vi "fuzzy_pid.vi"() -> ()   [LabVIEW 2019]
uses:
  <vilib>/addons/Fuzzy Logic/FL Fuzzy Controller (SISO).vi
  <vilib>/addons/Fuzzy Logic/NI_Fuzzy_Logic_API.lvlib
panel:
  in  "file path q2":path
  in  "file path q1":path
  out "Waveform Chart":T1(graph)
  in  "Set point":dbl
  in  "file path q0":path
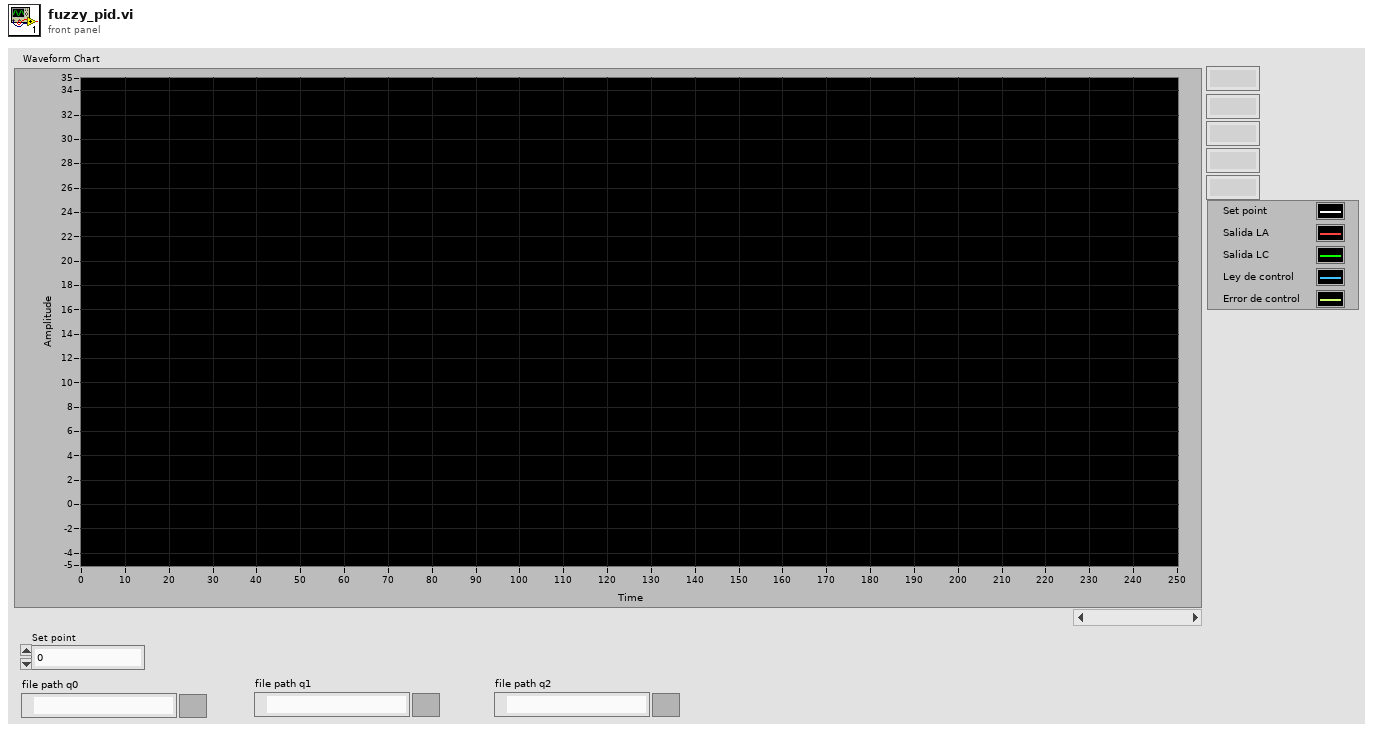
[diagram p1: front panel]
types:
  T1 = cluster{"Valvula (u_k)":dbl, "y_k":dbl, "y_k":dbl, dbl, dbl}
  T2 = typedef "NI_Fuzzy_Logic_API.lvlib/FL System.ctl" = cluster{"input variables":T3[], "output variables":T3[], "rules":T6[], "defuzzification method":T12, "description":string, "user MF interpolating polynomials":T13[]}
  T3 = typedef "NI_Fuzzy_Logic_API.lvlib/FL Variable.ctl" = cluster{"name":string, "range":dbl[], "MFs":T4[]}
  T4 = typedef "NI_Fuzzy_Logic_API.lvlib/FL Membership Function.ctl" = cluster{"name":string, "shape":T5, "points":dbl[], "color":u32, "user-defined shape index":i32}
  T5 = typedef "NI_Fuzzy_Logic_API.lvlib/FL Membership Function Shape.ctl" = u16
  T6 = typedef "NI_Fuzzy_Logic_API.lvlib/FL Rule.ctl" = cluster{"antecedents":T7[], "antecedent connective":T9, "consequents":T10[], "consequent implication":T11, "degree of support":dbl}
  T7 = typedef "NI_Fuzzy_Logic_API.lvlib/FL Antecedent.ctl" = cluster{"Var Index":i32, "MF Index":i32, "Cond":T8}
  T8 = typedef "NI_Fuzzy_Logic_API.lvlib/FL Modifier.ctl" = u16
  T9 = typedef "NI_Fuzzy_Logic_API.lvlib/FL Antecedent Connective.ctl" = u16
  T10 = typedef "NI_Fuzzy_Logic_API.lvlib/FL Consequent.ctl" = cluster{"Var Index":i32, "MF Index":i32, "Cond":T8}
  T11 = typedef "NI_Fuzzy_Logic_API.lvlib/FL Consequent Implication.ctl" = u16
  T12 = typedef "NI_Fuzzy_Logic_API.lvlib/FL Defuzzification.ctl" = u16
  T13 = typedef "NI_Fuzzy_Logic_API.lvlib/FL Interpolating polynomials.ctl" = cluster{"X":dbl[], "Y":dbl[], "Y(x) coeff":dbl[][], "X(y) coeff":dbl[][], "Area(y) coeff":dbl[][], "coa_x(y) coeff":dbl[][]}
  T14 = cluster{"Set point":dbl, "y_k":dbl, "y_k":dbl, dbl, dbl}
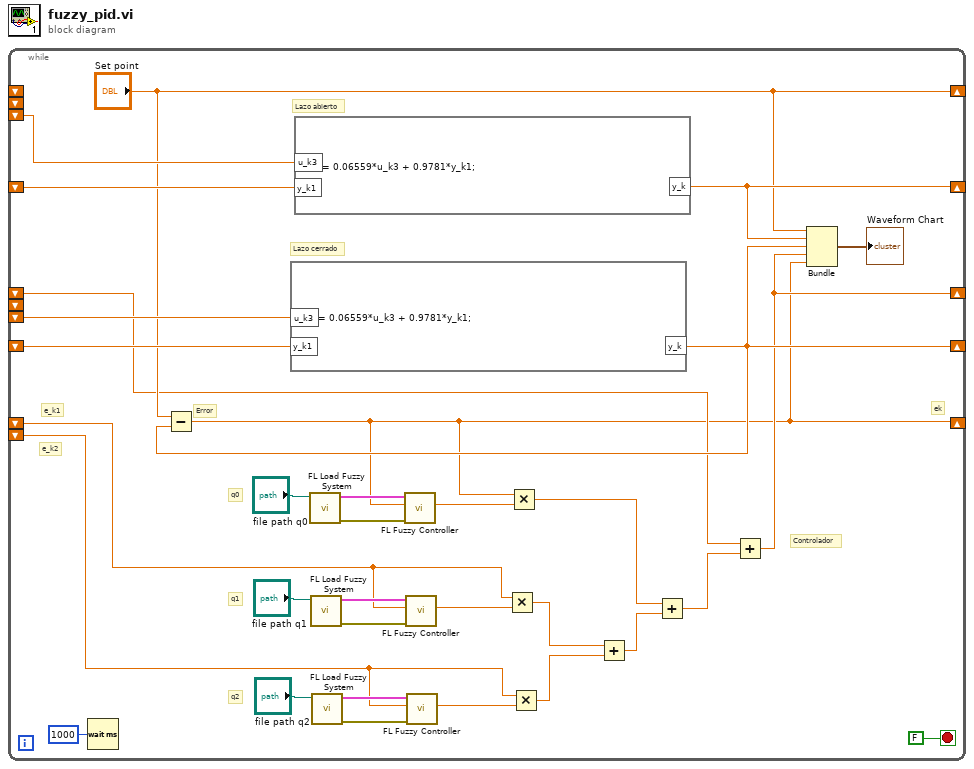
[diagram p0: block diagram]
diagram:
  n1 = while {
    shift-right: ["Set point"] -> _
    shift-left: _ -> [_]
    shift-left: _ -> [_]
    shift-left: _ -> [w32]
    shift-right: [w29] -> _
    shift-left: _ -> [w31]
    shift-right: [w21] -> _
    shift-left: _ -> [w24]
    shift-right: [w3] -> _
    shift-left: _ -> [w2]
    shift-left: _ -> [_]
    shift-left: _ -> [w23]
    shift-right: [w1] -> _
    shift-left: _ -> [w6]
    shift-left: _ -> [w5]
    stop <- FALSE stop-if-true
    # "Lazo cerrado"
    # "Lazo abierto"
    # "e_k2"
    # "e_k1"
    # "ek"
    # "Controlador"
    # "q2"
    # "q1"
    # "q0"
    # "Error"
    n2 = Wait (ms)(milliseconds to wait=u32 1000) -> ()  [unwired: 1 out]
    n3 = formula code="y_k = 0.06559*u_k3 + 0.9781*y_k1;"("u_k3"=w23, "y_k1"=w24) -> ("y_k"=w21:dbl)
    n4 = Subtract(x="Set point", y=w21) -> (x-y=w1:dbl)
    n5 = formula code="y_k = 0.06559*u_k3 + 0.9781*y_k1;"("u_k3"=w32, "y_k1"=w31) -> ("y_k"=w29:dbl)
    n6 = call <vilib>:"FL Load Fuzzy System.vi"("file path"="file path q0") -> ("error out"=w25:errorcluster, "fuzzy system out"=w26:T2)  [unwired: 9 in]
    n7 = call <vilib>:"FL Load Fuzzy System.vi"("file path"="file path q1") -> ("error out"=w18:errorcluster, "fuzzy system out"=w19:T2)  [unwired: 9 in]
    n8 = call <vilib>:"FL Load Fuzzy System.vi"("file path"="file path q2") -> ("error out"=w15:errorcluster, "fuzzy system out"=w16:T2)  [unwired: 9 in]
    n9 = call-poly <vilib>:"FL Fuzzy Controller.vi"("error in (no error)"=w25, "input value"=w1, "fuzzy system in"=w26) -> ("output value"=w7:dbl)  [unwired: 4 in, 4 out]
    n10 = call-poly <vilib>:"FL Fuzzy Controller.vi"("error in (no error)"=w18, "input value"=w6, "fuzzy system in"=w19) -> ("output value"=w9:dbl)  [unwired: 4 in, 4 out]
    n11 = call-poly <vilib>:"FL Fuzzy Controller.vi"("error in (no error)"=w15, "input value"=w5, "fuzzy system in"=w16) -> ("output value"=w8:dbl)  [unwired: 4 in, 4 out]
    n12 = Multiply(x=w6, y=w9) -> (x*y=w12:dbl)
    n13 = Multiply(x=w1, y=w7) -> (x*y=w10:dbl)
    n14 = Multiply(x=w5, y=w8) -> (x*y=w11:dbl)
    n15 = Add(x=w12, y=w11) -> (x+y=w13:dbl)
    n16 = Add(x=w10, y=w13) -> (x+y=w4:dbl)
    n17 = Add(x=w2, y=w4) -> (x+y=w3:dbl)
    n18 = Bundle("Set point"="Set point", "y_k"=w29, "y_k"=w21, w3, w1) -> (→"Waveform Chart":T14)  [unwired: 1 in]
  }
